vi "Main.vi"(11 "Module Admin":refnum<class "Delacor_lib_QMH_Module Admin.lvclass">) -> ()   [LabVIEW 2020, in "Hardware DAQ.lvlib"]
doc: "This template is based off of the Queued Message Handler design pattern and the Queued Message Handler project template that ships with LabVIEW.\n\nThe main difference is that the queue is private to this module and communication between modules is performed via Broadcast and Request events.\n\nRequest events are wrapped in public API methods and are handled in the Event Handling Loop (EHL) of this VI. Any module can register for Broadcast events sent by this module. The EHL generates messages based on user interface actions.\n\nThe Message Handling Loop (MHL) processes messages generated by the EHL, or by other messages. The messages are string values, so new messages can be added easily to the Message Cases case structure in the MHL. Each message cluster can also provide an optional value for Message Data, which is a variant that can be converted to whatever message-specific data is required.\n_____\nBased on DQMH Project Template 6.0.0.91."
uses:
  Hardware DAQ.lvlib
  <vilib>/Delacor/Delacor QMH/Libraries/Module Admin_class/Delacor_lib_QMH_Module Admin.lvclass
  Module Data--cluster.ctl
  <vilib>/Modbus/master/Modbus Master.lvclass
  Stop Argument--cluster.ctl
  <vilib>/Delacor/Delacor QMH/Libraries/Message Queue_class/Delacor_lib_QMH_Message Queue.lvclass/Delacor_lib_QMH_Message Queue.ctl
  <vilib>/Delacor/Delacor QMH/Libraries/Module Admin_class/Delacor_lib_QMH_Module Admin.lvclass/Delacor_lib_QMH_Module Admin.ctl
  Digital Output 0 Argument--cluster.ctl
  Digital Output 0 (Reply Payload)--cluster.ctl
  Digital Output 1 Argument--cluster.ctl
  Digital Output 1 (Reply Payload)--cluster.ctl
  Digital Output 2 Argument--cluster.ctl
  Digital Output 2 (Reply Payload)--cluster.ctl
  Digital Output 3 Argument--cluster.ctl
  Digital Output 3 (Reply Payload)--cluster.ctl
  <vilib>/Delacor/Delacor QMH/Libraries/Message Queue_class/Delacor_lib_QMH_Enqueue Message (Single).vi
  <vilib>/Delacor/Delacor QMH/Libraries/Module Admin_class/Delacor_lib_QMH_Get External Launch.vi
  <vilib>/DAQmx/read.llb/DAQmx Read (Analog 1D DBL NChan 1Samp).vi
  <vilib>/DAQmx/miscellaneous.llb/DAQmx Fill In Error Info.vi
  <vilib>/Utility/error.llb/Error Cluster From Error Code.vi
  <vilib>/ErrorRing/Error Ring.xnode
  <vilib>/Delacor/Delacor QMH/Libraries/Message Queue_class/Delacor_lib_QMH_Message Queue.lvclass
panel:
  out "Coil values":bool[](array[boolean])
  out "Estado de conexión":bool
  out "Volt":dbl[](array[numeric])
  in  "Update File ini":bool
  in  "Stop System":bool
  in  "Connected System":bool
  in  "Tab Control":enum32{"Adquisición", "Documentación"}(tab)
  out "PLC Logo":bool
  out "Xpress Board":bool
  out "Arduino UNO":bool
  out "NI - 9219":bool
  # "Sistema de Hadrware (DAQ)"
  # "DAQ - 9219"
  # "Arduino UNO"
  # "Xpress Board PIC"
  # "PLC Logo"
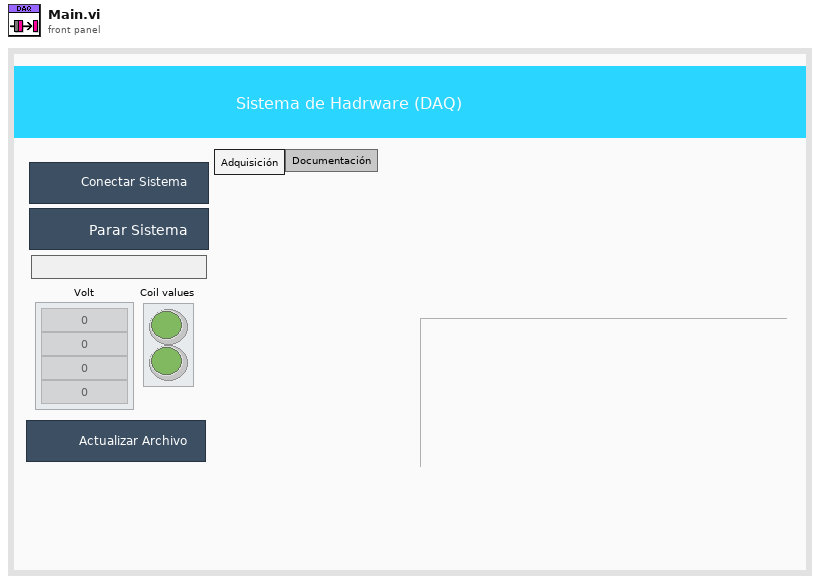
[diagram p1: front panel]
types:
  T1 = typedef "Hardware DAQ.lvlib/Request Events--cluster.ctl" = cluster{"Stop Module":refnum<user-event>, "Show Panel":refnum<user-event>, "Hide Panel":refnum<user-event>, "Get Module Execution Status":refnum<user-event>, "Show Diagram":refnum<user-event>, "Digital Output 0":refnum<user-event>, "Digital Output 1":refnum<user-event>, "Digital Output 2":refnum<user-event>, "Digital Output 3":refnum<user-event>}
  T2 = typedef "Hardware DAQ.lvlib/Module Data--cluster.ctl" = cluster{"File INI":cluster{"Hardware DAQ":cluster{"Hardware":string, "Puerto COM":string, "Task/channels in":string, "Direccion IP PLC":string, "Baudios":string, "Analog Input":string, "Digital Input":string, "Vref Max":string, "Resolución ADC Bits":string}}, "Comunication Hardware DAQ":cluster{"Hardware":enum16{"DAQ9219", "Arduino", "Xpress Board", "PLC Logo", "Default"}, "Status Connected?":bool, "Status File ini?":bool}, "Reference Hardware(s)":cluster{"task out":refnum<k21>, "VISA reference Port":refnum<visa-resource-name>, "TCP master instance":refnum<class "Modbus Master.lvclass">, "#AnalogInput":i32, "#DigitalInput":i32, "Vref Máx":i32, "Resolucion ADC Bits":i32}, "Data Process":cluster{"Volt":dbl[], "Volt DAQ NI9219":dbl[], "coil values":bool[]}}
  T3 = enum32{"invalid lock state", "Not Locked", "Locked (No Password)", "Password-protected"}
  T4 = typedef "Hardware DAQ.lvlib/Stop Argument--cluster.ctl" = cluster{"Origin":string, "Exit via Stop Module Req?":bool, "Wait for Module to stop?":bool}
  T5 = typedef "Hardware DAQ.lvlib/Digital Output 0 Argument--cluster.ctl" = cluster{"Digital Output 0":bool, "Wait Notifier":refnum<notifier>, "wait for reply":bool}
  T6 = typedef "Hardware DAQ.lvlib/Digital Output 1 Argument--cluster.ctl" = cluster{"Digital Output 1":bool, "Wait Notifier":refnum<notifier>, "wait for reply":bool}
  T7 = typedef "Hardware DAQ.lvlib/Digital Output 2 Argument--cluster.ctl" = cluster{"Digital Output 2":bool, "Wait Notifier":refnum<notifier>, "wait for reply":bool}
  T8 = typedef "Hardware DAQ.lvlib/Digital Output 3 Argument--cluster.ctl" = cluster{"Digital Output 3":bool, "Wait Notifier":refnum<notifier>, "wait for reply":bool}
  T9 = enum32{"Invalid", "Standard", "Closed", "Hidden", "Minimized", "Maximized"}
  T10 = enum16{"DAQ9219", "Arduino", "Xpress Board", "PLC Logo", "Default"}
  T11 = typedef "Hardware DAQ.lvlib/Digital Output 0 (Reply Payload)--cluster.ctl" = cluster{"Digital Output 0_I":bool, "error":errorcluster}
  T12 = typedef "Hardware DAQ.lvlib/Digital Output 1 (Reply Payload)--cluster.ctl" = cluster{"Digital Output 1_I":bool, "error":errorcluster}
  T13 = typedef "Hardware DAQ.lvlib/Digital Output 2 (Reply Payload)--cluster.ctl" = cluster{"Digital Output 2_I":bool, "error":errorcluster}
  T14 = typedef "Hardware DAQ.lvlib/Digital Output 3 (Reply Payload)--cluster.ctl" = cluster{"Digital Output 3_I":bool, "error":errorcluster}
  T15 = cluster{"Hardware":string, "Puerto COM":string, "Task/channels in":string, "Direccion IP PLC":string, "Baudios":string, "Analog Input":string, "Digital Input":string, "Vref Max":string, "Resolución ADC Bits":string}
  T16 = cluster{"#Analog Input":i32, "#Digital Input":i32, "Vref Máx":i32, "Resolucion ADC Bits":i32}
  T17 = cluster{"TCP master instance":refnum<class "Modbus Master.lvclass">, "VISA resource":refnum<visa-resource-name>, "task out":refnum<k21>}
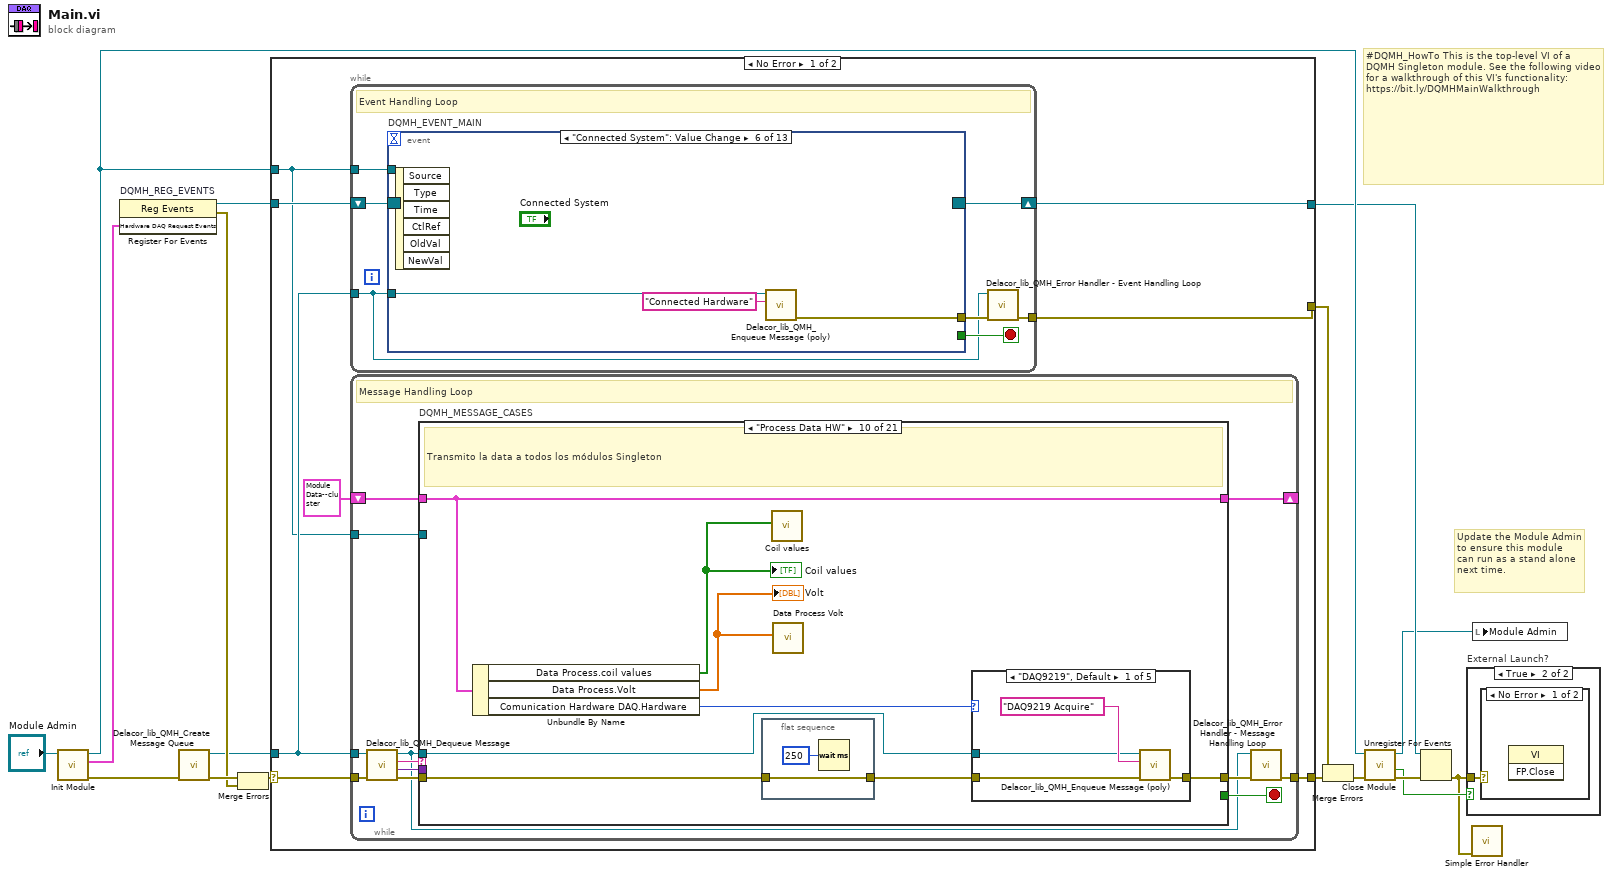
[diagram p0: block diagram]
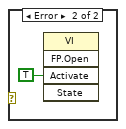
[diagram p3: hidden frame]
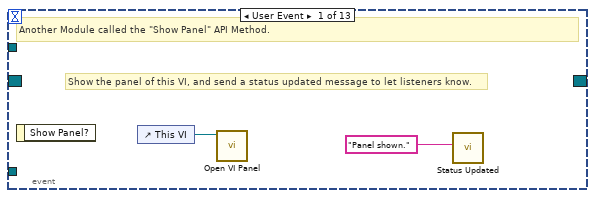
[diagram p4: hidden frame]
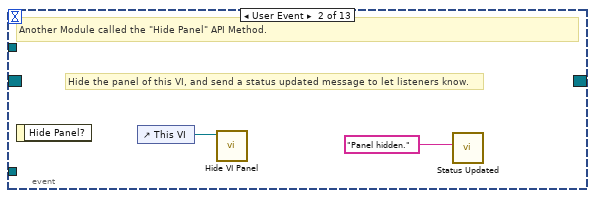
[diagram p5: hidden frame]
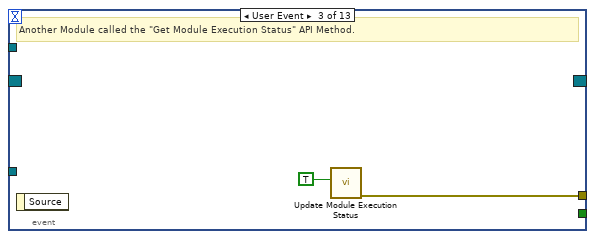
[diagram p6: hidden frame]
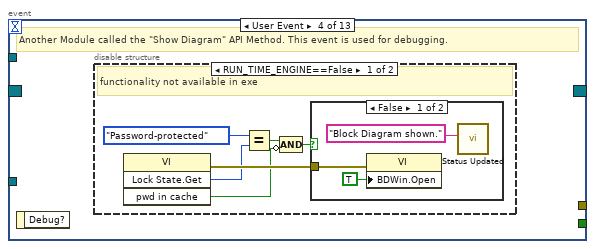
[diagram p7: hidden frame]
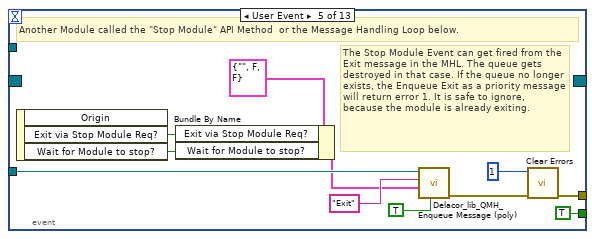
[diagram p10: hidden frame]
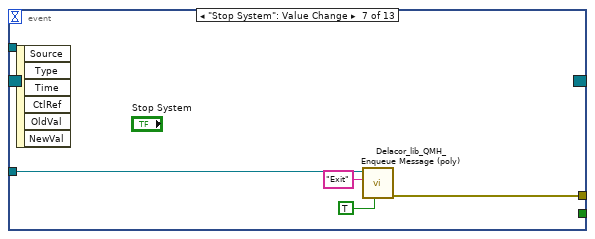
[diagram p11: hidden frame]
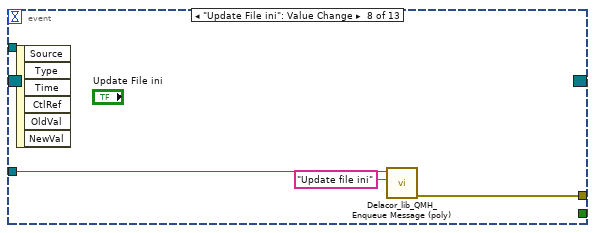
[diagram p12: hidden frame]
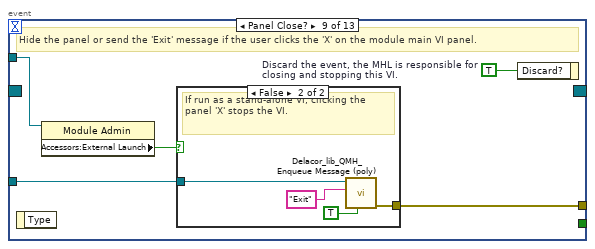
[diagram p13: hidden frame]
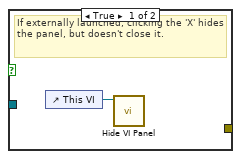
[diagram p14: hidden frame]
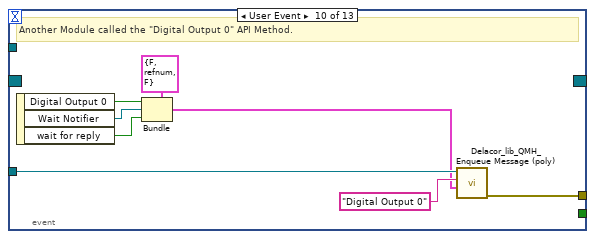
[diagram p15: hidden frame]
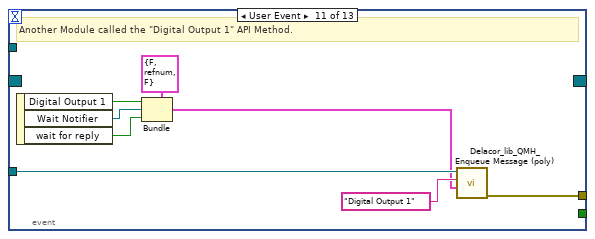
[diagram p16: hidden frame]
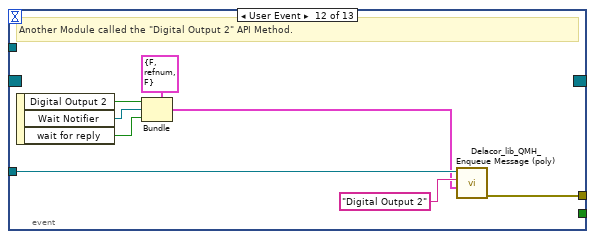
[diagram p17: hidden frame]
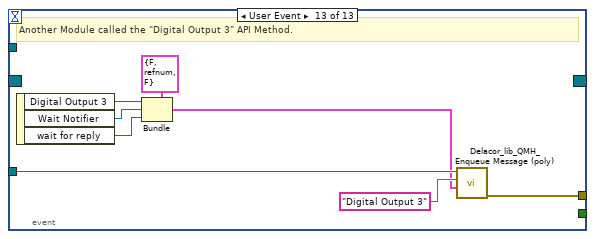
[diagram p18: hidden frame]
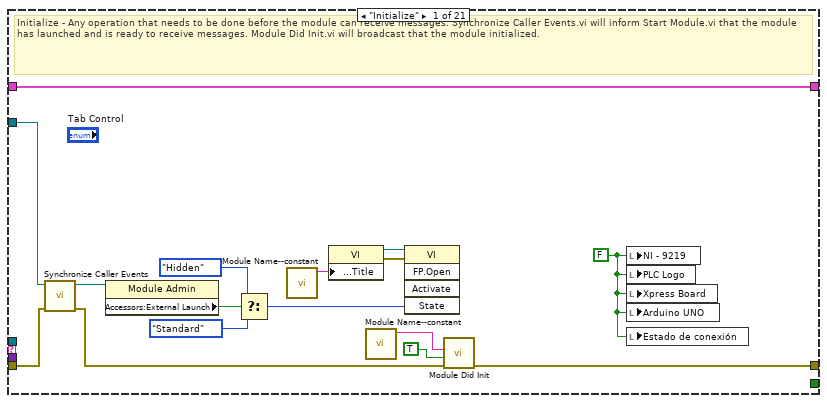
[diagram p19: hidden frame]
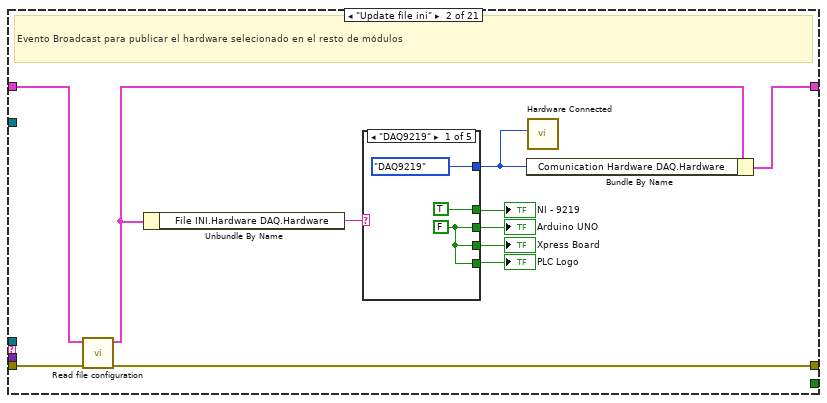
[diagram p20: hidden frame]
diagram:
  # "#DQMH_HowTo This is the top-level VI of a DQMH Singleton module. See the following video for a walkthrough of this VI's functionality: https://bit.ly/DQMHMainWalkthrough"
  # "Update the Module Admin to ensure this module can run as a stand alone next time."
  n1 = call "Init Module.vi"("Singleton Module Admin in"="Module Admin") -> ("error out"=w16:errorcluster, "Hardware DAQ Request Events"=w6:T1, "Singleton Module Admin out"=w9:refnum<class "Delacor_lib_QMH_Module Admin.lvclass">)  [unwired: 8 in]
  n2 = register-events "DQMH_REG_EVENTS"(w6) -> (reference out=w7:refnum<event-registration>, error out=w10:errorcluster)  [unwired: 2 in]
  n3 = call <vilib>:"Delacor_lib_QMH_Create Message Queue.vi"("error in"=w16) -> ("error out"=w12:errorcluster, "Message Queue"=w5:refnum<class "Delacor_lib_QMH_Message Queue.lvclass">)  [unwired: 9 in]
  n4 = Merge Errors(w12, w10) -> (w11:errorcluster)
  n5 = case shown="No Error" w11 {
    selector: w11 -> [w23 w588]
    tunnel: [w25 w587] -> w17
    tunnel: [w22 w593] -> w8
    tunnel: w7 -> [w20 w593]
    tunnel: w5 -> [w19 w586]
    tunnel: [w24 _] -> w14
    tunnel: w9 -> [w18 w589]
    frame No Error {
      n6 = while {
        tunnel: w19 -> [w26]
        shift-right: [w29] -> w22
        shift-left: w20 -> [w30]
        tunnel: [w31] -> w24
        tunnel: w18 -> [w27]
        stop <- w28 stop-if-true
        # "Event Handling Loop"
        n7 = event "DQMH_EVENT_MAIN" shown="[5] \"Connected System\": Value Change" {
          selector: w30 -> [_ _ _ _ _ _ _ _ _ _ _ _ _]
          dyn-events: [_ _ _ _ _ _ _ _ _ _ _ _ _] -> w29
          timeout: _ -> [_ _ _ _ _ _ _ _ _ _ _ _ _]
          tunnel: [_ _ _ _ TRUE ("Discard?") _ _ _ _ _ _ _ _] -> w28
          tunnel: w26 -> [_ _ _ _ w54 w60 w65 w67 w71 w86 w94 w102 w110]
          tunnel: [_ _ w38 _ w57 w61 w62 w68 w73 w79 w87 w95 w103] -> w32
          tunnel: w27 -> [_ _ _ _ _ _ _ _ w70 _ _ _ _]
          event User Event {
            # "Show the panel of this VI, and send a status updated message to let listeners know."
            # "Another Module called the \"Show Panel\" API Method."
            n8 = event-data() -> ()  [unwired: 1 in, 1 out]
            n9 = control-ref of="This VI"() -> (w34:refnum<vi>)
            n10 = call "Open VI Panel.vi"("VI"=w34) -> ()  [unwired: 10 in, 1 out]
            n11 = call "Status Updated.vi"("Status"="Panel shown." ("format string")) -> ()  [unwired: 10 in, 1 out]
          }
          event User Event {
            # "Hide the panel of this VI, and send a status updated message to let listeners know."
            # "Another Module called the \"Hide Panel\" API Method."
            n12 = event-data() -> ()  [unwired: 1 in, 1 out]
            n13 = control-ref of="This VI"() -> (w36:refnum<vi>)
            n14 = call "Hide VI Panel.vi"("VI"=w36) -> ()  [unwired: 10 in, 1 out]
            n15 = call "Status Updated.vi"("Status"="Panel hidden." ("format string")) -> ()  [unwired: 10 in, 1 out]
          }
          event User Event {
            # "Another Module called the \"Get Module Execution Status\" API Method."
            n16 = event-data() -> ()  [unwired: 1 in, 1 out]
            n17 = call "Update Module Execution Status.vi"("Running?"=TRUE) -> ("error out"=w38:errorcluster)  [unwired: 10 in]
          }
          event User Event {
            # "Another Module called the \"Show Diagram\" API Method. This event is used for debugging."
            n18 = event-data() -> ()  [unwired: 1 in, 1 out]
            n19 = disable-structure shown="RUN_TIME_ENGINE==False" {
              frame condition #0 (active) {
                # "functionality not available in exe"
                n20 = invoke class="VI" method="Lock State.Get"() -> (error out=w44:errorcluster, "Get Lock State"=w43:T3, "pwd in cache"=w40:bool)  [unwired: 4 in, 1 out]
                n21 = Equal?(x=T3."Password-protected", y=w43) -> (x = y?=w41:bool)
                n22 = Compound Arithmetic op=AND(w41, invert w40) -> (w39:bool)
                n23 = case shown="False" w39 {
                  tunnel: w44 -> [w47 _]
                  frame False {
                    n24 = property class="VI"(error in=w47, "BDWin.Open"=TRUE ("Block Diagram Window:Open")) -> ()  [unwired: 1 in, 2 out]
                    n25 = call "Status Updated.vi"("Status"="Block Diagram shown." ("format string")) -> ()  [unwired: 10 in, 1 out]
                  }
                  frame True {
                    # "Password-protected VI, and the password is not in the cache. Do not show the diagram."
                  }
                }
              }
              frame condition #1 {
              }
            }
          }
          event User Event {
            # "The Stop Module Event can get fired from the Exit message in the MHL. The queue gets destroyed in that case. If the queue no longer exists, the Enqueue Exit as a priority message will return error 1. It is safe to ignore, because the module is already exiting."
            # "Another Module called the \"Stop Module\" API Method  or the Message Handling Loop below."
            n26 = event-data() -> ("Exit via Stop Module Req?"=w50:bool, "Wait for Module to stop?"=w49:bool)  [unwired: 1 in, 1 out]
            n27 = Bundle By Name(cluster=T4 {"Origin"="", "Exit via Stop Module Req?"=FALSE, "Wait for Module to stop?"=FALSE} ("Stop Argument"), "Exit via Stop Module Req?"=w50, "Wait for Module to stop?"=w49) -> (w48:T4)
            n28 = call-poly <vilib>:"Delacor_lib_QMH_Enqueue Message (poly).vi"("Priority Message? (F)"=TRUE, "Message Data"=w48, "Message"="Exit", "Message Queue in"=w54) -> ("error out"=w58:errorcluster)  [unwired: 6 in, 1 out]
            n29 = call <vilib>:"Clear Errors.vi"("error in (no error)"=w58, "specific error code to clear (0: all)"=1) -> ("error out"=w57:errorcluster)  [unwired: 4 in, 1 out]
          }
          event "Connected System": Value Change {
            n30 = event-data() -> ()  [unwired: 1 in, 6 out]
            n31 = call-poly <vilib>:"Delacor_lib_QMH_Enqueue Message (poly).vi"("Message"="Connected Hardware", "Message Queue in"=w60) -> ("error out"=w61:errorcluster)  [unwired: 8 in, 1 out]
          }
          event "Stop System": Value Change {
            n32 = event-data() -> ()  [unwired: 1 in, 6 out]
            n33 = call-poly <vilib>:"Delacor_lib_QMH_Enqueue Message (poly).vi"("Priority Message? (F)"=TRUE, "Message"="Exit", "Message Queue in"=w65) -> ("error out"=w62:errorcluster)  [unwired: 7 in, 1 out]
          }
          event "Update File ini": Value Change {
            n34 = event-data() -> ()  [unwired: 1 in, 6 out]
            n35 = call-poly <vilib>:"Delacor_lib_QMH_Enqueue Message (poly).vi"("Message"="Update file ini", "Message Queue in"=w67) -> ("error out"=w68:errorcluster)  [unwired: 8 in, 1 out]
          }
          event Panel Close? {
            w72 = TRUE  # Discard the event, the MHL is responsible for closing and stopping this VI.
            # "Hide the panel or send the 'Exit' message if the user clicks the 'X' on the module main VI panel."
            n36 = event-data() -> ()  [unwired: 1 in, 1 out]
            n37 = property class="Module Admin"(reference=w70) -> ("Accessors:External Launch"=w69:bool)  [unwired: 1 in, 2 out]
            n38 = case shown="False" w69 {
              tunnel: w71 -> [_ w77]
              tunnel: [_ w78] -> w73
              frame True {
                # "If externally launched, clicking the 'X' hides the panel, but doesn't close it."
                n39 = control-ref of="This VI"() -> (w74:refnum<vi>)
                n40 = call "Hide VI Panel.vi"("VI"=w74) -> ()  [unwired: 10 in, 1 out]
              }
              frame False {
                # "If run as a stand-alone VI, clicking the panel 'X' stops the VI."
                n41 = call-poly <vilib>:"Delacor_lib_QMH_Enqueue Message (poly).vi"("Priority Message? (F)"=TRUE, "Message"="Exit", "Message Queue in"=w77) -> ("error out"=w78:errorcluster)  [unwired: 7 in, 1 out]
              }
            }
            n42 = event-data("Discard?"=w72) -> ()  [unwired: 1 in, 1 out]
          }
          event User Event {
            # "Another Module called the \"Digital Output 0\" API Method."
            n43 = event-data() -> ("Digital Output 0"=w82:bool, "Wait Notifier"=w81:refnum<notifier>, "wait for reply"=w80:bool)  [unwired: 1 in]
            n44 = Bundle(cluster=T5 {"Digital Output 0"=FALSE, "Wait Notifier"=refnum, "wait for reply"=FALSE} ("Digital Output 0 Argument"), "Digital Output 0"=w82, "Wait Notifier"=w81, "wait for reply"=w80) -> (w83:T5)
            n45 = call-poly <vilib>:"Delacor_lib_QMH_Enqueue Message (poly).vi"("Message Data"=w83, "Message"="Digital Output 0", "Message Queue in"=w86) -> ("error out"=w79:errorcluster)  [unwired: 7 in, 1 out]
          }
          event User Event {
            # "Another Module called the \"Digital Output 1\" API Method."
            n46 = event-data() -> ("Digital Output 1"=w90:bool, "Wait Notifier"=w89:refnum<notifier>, "wait for reply"=w88:bool)  [unwired: 1 in]
            n47 = Bundle(cluster=T6 {"Digital Output 1"=FALSE, "Wait Notifier"=refnum, "wait for reply"=FALSE} ("Digital Output 1 Argument"), "Digital Output 1"=w90, "Wait Notifier"=w89, "wait for reply"=w88) -> (w91:T6)
            n48 = call-poly <vilib>:"Delacor_lib_QMH_Enqueue Message (poly).vi"("Message Data"=w91, "Message"="Digital Output 1", "Message Queue in"=w94) -> ("error out"=w87:errorcluster)  [unwired: 7 in, 1 out]
          }
          event User Event {
            # "Another Module called the \"Digital Output 2\" API Method."
            n49 = event-data() -> ("Digital Output 2"=w98:bool, "Wait Notifier"=w97:refnum<notifier>, "wait for reply"=w96:bool)  [unwired: 1 in]
            n50 = Bundle(cluster=T7 {"Digital Output 2"=FALSE, "Wait Notifier"=refnum, "wait for reply"=FALSE} ("Digital Output 2 Argument"), "Digital Output 2"=w98, "Wait Notifier"=w97, "wait for reply"=w96) -> (w99:T7)
            n51 = call-poly <vilib>:"Delacor_lib_QMH_Enqueue Message (poly).vi"("Message Data"=w99, "Message"="Digital Output 2", "Message Queue in"=w102) -> ("error out"=w95:errorcluster)  [unwired: 7 in, 1 out]
          }
          event User Event {
            # "Another Module called the \"Digital Output 3\" API Method."
            n52 = event-data() -> ("Digital Output 3"=w106:bool, "Wait Notifier"=w105:refnum<notifier>, "wait for reply"=w104:bool)  [unwired: 1 in]
            n53 = Bundle(cluster=T8 {"Digital Output 3"=FALSE, "Wait Notifier"=refnum, "wait for reply"=FALSE} ("Digital Output 3 Argument"), "Digital Output 3"=w106, "Wait Notifier"=w105, "wait for reply"=w104) -> (w107:T8)
            n54 = call-poly <vilib>:"Delacor_lib_QMH_Enqueue Message (poly).vi"("Message Data"=w107, "Message"="Digital Output 3", "Message Queue in"=w110) -> ("error out"=w103:errorcluster)  [unwired: 7 in, 1 out]
          }
        }
        n55 = call-dynamic "Delacor_lib_QMH_Error Handler - Event Handling Loop.vi"("error in"=w32, "Message Queue in"=w26) -> ("dup error in"=w31:errorcluster)  [unwired: 8 in, 1 out]
      }
      n56 = while {
        tunnel: w19 -> [w113]
        shift-right: [w117] -> _
        shift-left: T2 {"File INI"={"Hardware DAQ"={"Hardware"="", "Puerto COM"="", "Task/channels in"="", "Direccion IP PLC"="", "Baudios"="", "Analog Input"="", "Digital Input"="", "Vref Max"="", "Resolución ADC Bits"=""}}, "Comunication Hardware DAQ"={"Hardware"=enum."DAQ9219", "Status Connected?"=FALSE, "Status File ini?"=FALSE}, "Reference Hardware(s)"={"task out"="", "VISA reference Port"="", "TCP master instance"=refnum, "#AnalogInput"=0, "#DigitalInput"=0, "Vref Máx"=0, "Resolucion ADC Bits"=0}, "Data Process"={"Volt"=[], "Volt DAQ NI9219"=[], "coil values"=[]}} ("Data Cluster") -> [w118]
        tunnel: w23 -> [w121]
        tunnel: [w119] -> w25
        tunnel: w18 -> [w111]
        stop <- w116 stop-if-true
        # "Message Handling Loop"
        n57 = call-dynamic "Delacor_lib_QMH_Dequeue Message.vi"("error in"=w121, "Message Queue in"=w113) -> ("error out"=w120:errorcluster, "Message Data"=w114:variant, "Message"=w115:string, "Message Queue out"=w112:refnum<class "Delacor_lib_QMH_Message Queue.lvclass">)  [unwired: 6 in]
        n58 = case "DQMH_MESSAGE_CASES" shown="\"Process Data HW\"" w115 {
          selector: w115 -> [_ _ _ _ _ _ _ _ _ _ _ _ _ _ _ _ _ _ _ _ w573]
          tunnel: w112 -> [_ _ w179 w187 w208 w221 w251 w278 w284 w298 _ _ _ _ _ _ _ _ w540 w566 _]
          tunnel: w120 -> [w137 w149 w178 w185 w216 w227 w257 w280 w294 w299 w323 w342 w391 w440 w489 w522 w524 w529 w546 w571 w575]
          tunnel: [w135 w139 w180 w186 w207 w220 w250 w279 w283 w297 w323 w328 w374 w422 w471 w521 w524 w528 w537 w568 w576] -> w122
          tunnel: w118 -> [w124 w148 w183 w189 w215 w231 w261 w282 w290 w302 w322 w330 w383 w432 w481 w520 w523 w526 w542 w554 w574]
          tunnel: [w124 w145 w182 w189 w211 w222 w252 w282 w287 w302 w322 w327 w382 w431 w480 w520 w523 w526 w542 w554 w574] -> w117
          tunnel: [_ _ _ _ _ _ _ _ _ _ _ _ _ _ _ _ _ _ _ w565 _] -> w116
          tunnel: w114 -> [_ _ _ _ _ _ _ _ _ _ _ w341 w390 w439 w488 _ _ _ w541 w564 _]
          tunnel: w111 -> [w128 _ _ _ _ _ _ _ _ _ _ _ _ _ _ _ _ _ w539 w559 _]
          frame "Initialize" {
            w123 = FALSE ("PLC Logo")
            # "Initialize - Any operation that needs to be done before the module can receive messages. Synchronize Caller Events.vi will inform Start Module.vi that the module has launched and is ready to receive messages. Module Did Init.vi will broadcast that the module initialized."
            n59 = call "Synchronize Caller Events.vi"("error in (no error)"=w137, "Singleton Module Admin in"=w128) -> ("error out"=w136:errorcluster, "Singleton Module Admin out"=w125:refnum<class "Delacor_lib_QMH_Module Admin.lvclass">)  [unwired: 8 in]
            n60 = property class="Module Admin"(reference=w125) -> ("Accessors:External Launch"=w132:bool)  [unwired: 1 in, 2 out]
            n61 = Select(t=T9."Hidden" ("State"), s=w132, f=T9."Standard" ("State")) -> (s? t:f=w129:T9)
            n62 = call "Module Name--constant.vi"() -> ("Module Name"=w134:string)  [unwired: 11 in]
            n63 = property class="VI"("Front Panel.Title"=w134) -> (reference out=w133:refnum<vi>, error out=w138:errorcluster)  [unwired: 2 in]
            n64 = call "Module Name--constant.vi"() -> ("Module Name"=w126:string)  [unwired: 11 in]
            n65 = invoke class="VI" method="FP.Open"(reference=w133, error in=w138, "State"=w129) -> ()  [unwired: 2 in, 5 out]
            n66 = call "Module Did Init.vi"("error in (no error)"=w136, "Initialized?"=TRUE, "Origin"=w126) -> ("error out"=w135:errorcluster)  [unwired: 8 in]
            n67 = local write "NI - 9219"(w123) -> ()
            n68 = local write "PLC Logo"(w123) -> ()
            n69 = local write "Xpress Board"(w123) -> ()
            n70 = local write "Arduino UNO"(w123) -> ()
            n71 = local write "Estado de conexión"(w123) -> ()
          }
          frame "Update file ini" {
            # "Evento Broadcast para publicar el hardware selecionado en el resto de módulos"
            n72 = call "Read file configuration.vi"("error in (no error)"=w149, "Data Cluster"=w148) -> ("error out"=w139:errorcluster, "Data Cluster out"=w146:T2)  [unwired: 8 in]
            n73 = Unbundle By Name(w146) -> ("File INI.Hardware DAQ.Hardware"=w147:string)
            n74 = case shown="\"DAQ9219\"" w147 {
              tunnel: [TRUE ("NI - 9219") w154 w157 w160 w163] -> w143
              tunnel: [w151 TRUE ("Arduino UNO") w157 w160 w163] -> w142
              tunnel: [w151 w154 TRUE ("Arduino UNO") w160 w163] -> w141
              tunnel: [w151 w154 w157 TRUE ("Arduino UNO") w163] -> w140
              tunnel: [T10."DAQ9219" T10."Arduino" T10."Xpress Board" T10."PLC Logo" T10."Default"] -> w144
              frame "DAQ9219" {
                w151 = FALSE ("Arduino UNO")
              }
              frame "Arduino" {
                w154 = FALSE ("NI - 9219")
              }
              frame "Xpress Board" {
                w157 = FALSE ("NI - 9219")
              }
              frame "PLC" {
                w160 = FALSE ("NI - 9219")
              }
              frame "Default", Default {
                w163 = FALSE ("NI - 9219")
              }
            }
            "NI - 9219" <- w143
            "Arduino UNO" <- w142
            "Xpress Board" <- w141
            "PLC Logo" <- w140
            n75 = Bundle By Name(cluster=w146, "Comunication Hardware DAQ.Hardware"=w144) -> (w145:T2)
            n76 = call "Hardware Connected.vi"("Hardware Connected"=w144) -> ()  [unwired: 10 in, 1 out]
          }
          frame "Connected Hardware" {
            n77 = Unbundle By Name(w183) -> ("File INI.Hardware DAQ"=w176:T15, "Comunication Hardware DAQ.Hardware"=w177:T10)
            n78 = call "Select Hardware.vi"("error in (no error)"=w178, "Hardware"=w177, "File INI.Hardware DAQ"=w176) -> ("error out"=w164:errorcluster, "#Parametros HW"=w171:T16, "Reference HW"=w175:T17)  [unwired: 6 in]
            n79 = Unbundle By Name(w171) -> ("#Analog Input"=w170:i32, "#Digital Input"=w169:i32, "Vref Máx"=w168:i32, "Resolucion ADC Bits"=w167:i32)
            n80 = Unbundle By Name(w175) -> ("TCP master instance"=w174:refnum<class "Modbus Master.lvclass">, "task out"=w173:refnum<k21>, "VISA resource"=w172:refnum<visa-resource-name>)
            n81 = Unbundle By Name(w164) -> ("status"=w166:bool)
            n82 = Not(x=w166) -> (.not. x?=w165:bool)
            n83 = Bundle By Name(cluster=w183, "Reference Hardware(s).TCP master instance"=w174, "Reference Hardware(s).task out"=w173, "Reference Hardware(s).VISA reference Port"=w172, "Reference Hardware(s).#AnalogInput"=w170, "Reference Hardware(s).#DigitalInput"=w169, "Reference Hardware(s).Vref Máx"=w168, "Reference Hardware(s).Resolucion ADC Bits"=w167, "Comunication Hardware DAQ.Status Connected?"=w165) -> (w182:T2)
            n84 = call-poly <vilib>:"Delacor_lib_QMH_Enqueue Message (poly).vi"("error in"=w164, "Message"="Update HMI User", "Message Queue in"=w179) -> ("error out"=w180:errorcluster)  [unwired: 7 in, 1 out]
          }
          frame "Update HMI User" {
            n85 = Unbundle By Name(w189) -> ("Comunication Hardware DAQ.Status Connected?"=→"Estado de conexión":bool, "Comunication Hardware DAQ.Hardware"=w188:T10)
            n86 = case shown="\"DAQ9219\", Default" w188 {
              tunnel: w187 -> [w192 w196 w200 w204 _]
              tunnel: [w191 w195 w199 w203 w206] -> w186
              tunnel: w185 -> [w190 w194 w198 w202 w206]
              frame "DAQ9219", Default {
                n87 = call-poly <vilib>:"Delacor_lib_QMH_Enqueue Message (poly).vi"("error in"=w190, "Message"="DAQ9219 Acquire", "Message Queue in"=w192) -> ("error out"=w191:errorcluster)  [unwired: 7 in, 1 out]
              }
              frame "Arduino" {
                n88 = call-poly <vilib>:"Delacor_lib_QMH_Enqueue Message (poly).vi"("error in"=w194, "Message"="Arduino Acquire", "Message Queue in"=w196) -> ("error out"=w195:errorcluster)  [unwired: 7 in, 1 out]
              }
              frame "Xpress Board" {
                n89 = call-poly <vilib>:"Delacor_lib_QMH_Enqueue Message (poly).vi"("error in"=w198, "Message"="Xpress Board Acquire", "Message Queue in"=w200) -> ("error out"=w199:errorcluster)  [unwired: 7 in, 1 out]
              }
              frame "PLC Logo" {
                n90 = call-poly <vilib>:"Delacor_lib_QMH_Enqueue Message (poly).vi"("error in"=w202, "Message"="PLC Acquire", "Message Queue in"=w204) -> ("error out"=w203:errorcluster)  [unwired: 7 in, 1 out]
              }
              frame "Default" {
              }
            }
          }
          frame "DAQ9219 Acquire" {
            n91 = Unbundle By Name(w215) -> ("Reference Hardware(s).task out"=w217:refnum<k21>)
            n92 = call-poly <vilib>:"DAQmx Read.vi"("task/channels in"=w217, "timeout"=1000.0, "error in"=w216) -> ("task out"=w214:refnum<k21>, "data"=w213:dbl[], "error out"=w209:errorcluster)  [unwired: 10 in]
            n93 = Bundle By Name(cluster=w215, "Reference Hardware(s).task out"=w214, "Data Process.Volt"=w213) -> (w211:T2)
            n94 = call-poly <vilib>:"Delacor_lib_QMH_Enqueue Message (poly).vi"("error in"=w209, "Message"="Process Data HW", "Message Queue in"=w208) -> ("error out"=w207:errorcluster)  [unwired: 7 in, 1 out]
          }
          frame "Arduino Acquire" {
            w226 = enum16{"AI-0", "AI-1", "AI-2", "AI-3"}[] [enum."AI-0", enum."AI-1", enum."AI-2", enum."AI-3"] items=["AI-0", "AI-1", "AI-2", "AI-3"]
            n95 = Unbundle By Name(w231) -> ("Reference Hardware(s).VISA reference Port"=w230:refnum<visa-resource-name>, "Reference Hardware(s).#AnalogInput"=w225:i32, "Reference Hardware(s).Vref Máx"=w229:i32, "Reference Hardware(s).Resolucion ADC Bits"=w228:i32)  [unwired: 1 out]
            n96 = for {
              N: w225 -> [_]
              tunnel: w230 -> [w247]
              tunnel: w229 -> [w244]
              tunnel: w228 -> [w243]
              tunnel: w227 -> [w246]
              tunnel: w226 -> [w245] mode=indexing
              tunnel: [w242] -> w218
              tunnel: [w241] -> w224
              tunnel: [w240] -> w223 mode=indexing
              n97 = call "Read Analog Input.vi"("VISA Refnum in"=w247, "#Pin analogico"=w245, "Vref Máx"=w244, "Resolucion ADC Bits"=w243, "error in (no error)"=w246) -> ("VISA Refnum out"=w241:refnum<visa-resource-name>, "Volt"=w240:dbl, "error out"=w242:errorcluster)  [unwired: 8 in]
            }
            n98 = Unbundle By Name(w218) -> ("code"=w219:i32)
            n99 = Bundle By Name(cluster=w231, "Reference Hardware(s).VISA reference Port"=w224, "Data Process.Volt"=w223) -> (w222:T2)
            n100 = case shown="1023" w219 {
              tunnel: w221 -> [w232 w238]
              tunnel: [w233 w237] -> w220
              tunnel: w218 -> [w234 w236]
              frame 1023 {
                n101 = call-poly <vilib>:"Delacor_lib_QMH_Enqueue Message (poly).vi"("error in"=w234, "Message"="Exit", "Message Queue in"=w232) -> ("error out"=w233:errorcluster)  [unwired: 7 in, 1 out]
              }
              frame 1, Default {
                n102 = call-poly <vilib>:"Delacor_lib_QMH_Enqueue Message (poly).vi"("error in"=w236, "Message"="Process Data HW", "Message Queue in"=w238) -> ("error out"=w237:errorcluster)  [unwired: 7 in, 1 out]
              }
            }
          }
          frame "Xpress Board Acquire" {
            w256 = enum16{"AI-0", "AI-1", "AI-2", "AI-3"}[] [enum."AI-0", enum."AI-1", enum."AI-2", enum."AI-3"] items=["AI-0", "AI-1", "AI-2", "AI-3"]
            n103 = Unbundle By Name(w261) -> ("Reference Hardware(s).VISA reference Port"=w260:refnum<visa-resource-name>, "Reference Hardware(s).#AnalogInput"=w255:i32, "Reference Hardware(s).Vref Máx"=w259:i32, "Reference Hardware(s).Resolucion ADC Bits"=w258:i32)  [unwired: 1 out]
            n104 = for {
              N: w255 -> [_]
              tunnel: w260 -> [w277]
              tunnel: w259 -> [w274]
              tunnel: w258 -> [w273]
              tunnel: w257 -> [w276]
              tunnel: w256 -> [w275] mode=indexing
              tunnel: [w272] -> w248
              tunnel: [w271] -> w254
              tunnel: [w270] -> w253 mode=indexing
              n105 = call "Read Analog Input.vi"("VISA Refnum in"=w277, "#Pin analogico"=w275, "Vref Máx"=w274, "Resolucion ADC Bits"=w273, "error in (no error)"=w276) -> ("VISA Refnum out"=w271:refnum<visa-resource-name>, "Volt"=w270:dbl, "error out"=w272:errorcluster)  [unwired: 8 in]
            }
            n106 = Unbundle By Name(w248) -> ("code"=w249:i32)
            n107 = Bundle By Name(cluster=w261, "Reference Hardware(s).VISA reference Port"=w254, "Data Process.Volt"=w253) -> (w252:T2)
            n108 = case shown="Default" w249 {
              tunnel: w251 -> [w262 w268]
              tunnel: [w263 w267] -> w250
              tunnel: w248 -> [w264 w266]
              frame 1023 {
                n109 = call-poly <vilib>:"Delacor_lib_QMH_Enqueue Message (poly).vi"("error in"=w264, "Message"="Exit", "Message Queue in"=w262) -> ("error out"=w263:errorcluster)  [unwired: 7 in, 1 out]
              }
              frame Default {
                n110 = call-poly <vilib>:"Delacor_lib_QMH_Enqueue Message (poly).vi"("error in"=w266, "Message"="Process Data HW", "Message Queue in"=w268) -> ("error out"=w267:errorcluster)  [unwired: 7 in, 1 out]
              }
            }
          }
          frame "PLC Acquire" {
            n111 = call-poly <vilib>:"Delacor_lib_QMH_Enqueue Message (poly).vi"("error in"=w280, "Message"="Read Digital Inputs", "Message Queue in"=w278) -> ("error out"=w279:errorcluster)  [unwired: 7 in, 1 out]
          }
          frame "Read Digital Inputs" {
            n112 = Unbundle By Name(w290) -> ("Reference Hardware(s).TCP master instance"=w293:refnum<class "Modbus Master.lvclass">)
            n113 = call-dynamic "Read Coils.vi"("error in (no error)"=w294, "number of coils"=u16 4, "starting address"=u16 0, "Modbus master in"=w293) -> ("error out"=w285:errorcluster, "coil values"=w288:bool[], "Modbus master out"=w289:refnum<class "Modbus Master.lvclass">)  [unwired: 5 in]
            n114 = Bundle By Name(cluster=w290, "Reference Hardware(s).TCP master instance"=w289, "Data Process.coil values"=w288) -> (w287:T2)
            n115 = call-poly <vilib>:"Delacor_lib_QMH_Enqueue Message (poly).vi"("error in"=w285, "Message"="Process Data HW", "Message Queue in"=w284) -> ("error out"=w283:errorcluster)  [unwired: 7 in, 1 out]
          }
          frame "Process Data HW" {
            # "Transmito la data a todos los módulos Singleton"
            n116 = Unbundle By Name(w302) -> ("Data Process.coil values"=w295:bool[], "Data Process.Volt"=w296:dbl[], "Comunication Hardware DAQ.Hardware"=w301:T10)
            "Volt" <- w296
            "Coil values" <- w295
            n117 = flat-sequence {
              tunnel: [w304] -> w300
              tunnel: w299 -> [w304]
              frame #0 {
                n118 = Wait (ms)(milliseconds to wait=u32 250) -> ()  [unwired: 1 out]
              }
            }
            n119 = call "Coil values.vi"("Data Process.coil values"=w295) -> ()  [unwired: 10 in, 1 out]
            n120 = call "Data Process Volt.vi"("Data Process.Volt"=w296) -> ()  [unwired: 10 in, 1 out]
            n121 = case shown="\"DAQ9219\", Default" w301 {
              tunnel: w298 -> [w307 w311 w315 w319 _]
              tunnel: [w306 w310 w314 w318 w321] -> w297
              tunnel: w300 -> [w305 w309 w313 w317 w321]
              frame "DAQ9219", Default {
                n122 = call-poly <vilib>:"Delacor_lib_QMH_Enqueue Message (poly).vi"("error in"=w305, "Message"="DAQ9219 Acquire", "Message Queue in"=w307) -> ("error out"=w306:errorcluster)  [unwired: 7 in, 1 out]
              }
              frame "Arduino" {
                n123 = call-poly <vilib>:"Delacor_lib_QMH_Enqueue Message (poly).vi"("error in"=w309, "Message"="Arduino Acquire", "Message Queue in"=w311) -> ("error out"=w310:errorcluster)  [unwired: 7 in, 1 out]
              }
              frame "Xpress Board" {
                n124 = call-poly <vilib>:"Delacor_lib_QMH_Enqueue Message (poly).vi"("error in"=w313, "Message"="Xpress Board Acquire", "Message Queue in"=w315) -> ("error out"=w314:errorcluster)  [unwired: 7 in, 1 out]
              }
              frame "PLC Logo" {
                n125 = call-poly <vilib>:"Delacor_lib_QMH_Enqueue Message (poly).vi"("error in"=w317, "Message"="PLCAcquire", "Message Queue in"=w319) -> ("error out"=w318:errorcluster)  [unwired: 7 in, 1 out]
              }
              frame "Default" {
              }
            }
          }
          frame "---Module Specific---" {
            # "Separator -- The following cases handle messages specific to this Module."
          }
          frame "Digital Output 0" {
            # "Digital Output 0 to Hardware"
            n126 = Variant To Data(error in=w342, type=T5 {"Digital Output 0"=FALSE, "Wait Notifier"=refnum, "wait for reply"=FALSE} ("Digital Output 0 Argument"), Variant=w341) -> (data=w339:T5, error out=w334:errorcluster)
            n127 = Unbundle By Name(w330) -> ("Reference Hardware(s).TCP master instance"=w325:refnum<class "Modbus Master.lvclass">, "Reference Hardware(s).VISA reference Port"=w333:refnum<visa-resource-name>, "Comunication Hardware DAQ.Hardware"=w326:T10)
            n128 = Unbundle By Name(w339) -> ("Digital Output 0"=w332:bool, "Wait Notifier"=w338:refnum<notifier>, "wait for reply"=w337:bool)
            n129 = case shown="\"Xpress Board\"" w326 {
              tunnel: w334 -> [w346 w354 w362 w370]
              tunnel: w333 -> [w344 w353 w361 w363]
              tunnel: w332 -> [w345 w351 w359 w369]
              tunnel: [w345 w350 w358 w364] -> w331
              tunnel: [w344 w349 w357 w363] -> w329
              tunnel: [w346 w348 w356 w366] -> w328
              tunnel: w325 -> [w343 w347 w355 w368]
              tunnel: [w343 w347 w355 w365] -> w324
              frame "DAQ9219", Default {
                # "No hay nada"
              }
              frame "Arduino" {
                n130 = call "Write Digital Output.vi"("error in (no error)"=w354, "State"=w351, "#Pin Digital Out"=enum16{"DO-0", "DO-1", "DO-2", "DO-3"}."DO-0", "VISA reference in"=w353) -> ("error out"=w348:errorcluster, "State dispare?"=w350:bool, "VISA reference out"=w349:refnum<visa-resource-name>)  [unwired: 5 in]
              }
              frame "Xpress Board" {
                n131 = call "Write Digital Output.vi"("error in (no error)"=w362, "State"=w359, "#Pin Digital Out"=enum16{"DO-0", "DO-1", "DO-2", "DO-3"}."DO-0", "VISA reference in"=w361) -> ("error out"=w356:errorcluster, "State dispare?"=w358:bool, "VISA reference out"=w357:refnum<visa-resource-name>)  [unwired: 5 in]
              }
              frame "PLC Logo" {
                n132 = call "Digital Output 0-10V.vi"("error in (no error)"=w370, "State"=w369, "#Pin 0-10V"=enum16{"DO-0", "DO-1", "DO-2", "DO-3"}."DO-0", "Modbus Master in"=w368) -> ("error out"=w366:errorcluster, "State Send?"=w364:bool, "Modbus master out"=w365:refnum<class "Modbus Master.lvclass">)  [unwired: 5 in]
              }
            }
            n133 = Bundle By Name(cluster=w330, "Reference Hardware(s).TCP master instance"=w324, "Reference Hardware(s).VISA reference Port"=w329) -> (w327:T2)
            n134 = Bundle By Name(cluster=T11 {"Digital Output 0_I"=FALSE, "error"={"status"=FALSE, "code"=0, "source"=""}} ("Digital Output 0 (Reply Payload)"), "Digital Output 0_I"=w331, "error"=w328) -> (w336:T11)
            n135 = case shown="True" w337 {
              tunnel: w338 -> [_ w372]
              tunnel: w336 -> [_ w371]
              frame False {
              }
              frame True {
                n136 = Send Notification(notification=w371, notifier=w372) -> ()  [unwired: 1 in, 2 out]
              }
            }
          }
          frame "Digital Output 1" {
            # "Digital Output 1 to Hardware"
            n137 = Variant To Data(error in=w391, type=T6 {"Digital Output 1"=FALSE, "Wait Notifier"=refnum, "wait for reply"=FALSE} ("Digital Output 1 Argument"), Variant=w390) -> (data=w388:T6, error out=w381:errorcluster)
            n138 = Unbundle By Name(w383) -> ("Reference Hardware(s).TCP master instance"=w378:refnum<class "Modbus Master.lvclass">, "Reference Hardware(s).VISA reference Port"=w379:refnum<visa-resource-name>, "Comunication Hardware DAQ.Hardware"=w380:T10)
            n139 = Unbundle By Name(w388) -> ("Digital Output 1"=w373:bool, "Wait Notifier"=w387:refnum<notifier>, "wait for reply"=w386:bool)
            n140 = case shown="\"PLC Logo\"" w380 {
              tunnel: [FALSE ("State Send?") w402 w410 w416] -> w375
              tunnel: [w393 w401 w409 w413] -> w376
              tunnel: [w395 w400 w408 w418] -> w374
              tunnel: [w392 w399 w405 w417] -> w377
              tunnel: w381 -> [w395 w398 w407 w415]
              tunnel: w379 -> [w393 w396 w406 w413]
              tunnel: w378 -> [w392 w399 w405 w412]
              tunnel: w373 -> [_ w397 w404 w414]
              frame "DAQ9219", Default {
                # "No hay nada"
              }
              frame "Arduino" {
                n141 = call "Write Digital Output.vi"("error in (no error)"=w398, "State"=w397, "#Pin Digital Out"=enum16{"DO-0", "DO-1", "DO-2", "DO-3"}."DO-1", "VISA reference in"=w396) -> ("error out"=w400:errorcluster, "State dispare?"=w402:bool, "VISA reference out"=w401:refnum<visa-resource-name>)  [unwired: 5 in]
              }
              frame "Xpress Board" {
                n142 = call "Write Digital Output.vi"("error in (no error)"=w407, "State"=w404, "#Pin Digital Out"=enum16{"DO-0", "DO-1", "DO-2", "DO-3"}."DO-1", "VISA reference in"=w406) -> ("error out"=w408:errorcluster, "State dispare?"=w410:bool, "VISA reference out"=w409:refnum<visa-resource-name>)  [unwired: 5 in]
              }
              frame "PLC Logo" {
                n143 = call "Digital Output 0-10V.vi"("error in (no error)"=w415, "State"=w414, "#Pin 0-10V"=enum16{"DO-0", "DO-1", "DO-2", "DO-3"}."DO-1", "Modbus Master in"=w412) -> ("error out"=w418:errorcluster, "State Send?"=w416:bool, "Modbus master out"=w417:refnum<class "Modbus Master.lvclass">)  [unwired: 5 in]
              }
            }
            n144 = Bundle By Name(cluster=w383, "Reference Hardware(s).TCP master instance"=w377, "Reference Hardware(s).VISA reference Port"=w376) -> (w382:T2)
            n145 = Bundle By Name(cluster=T12 {"Digital Output 1_I"=FALSE, "error"={"status"=FALSE, "code"=0, "source"=""}} ("Digital Output 1 (Reply Payload)"), "Digital Output 1_I"=w375, "error"=w374) -> (w385:T12)
            n146 = case shown="True" w386 {
              tunnel: w387 -> [_ w421]
              tunnel: w385 -> [_ w420]
              frame False {
              }
              frame True {
                n147 = Send Notification(notification=w420, notifier=w421) -> ()  [unwired: 1 in, 2 out]
              }
            }
          }
          frame "Digital Output 2" {
            # "Digital Output 2 to Hardware"
            n148 = Variant To Data(error in=w440, type=T7 {"Digital Output 2"=FALSE, "Wait Notifier"=refnum, "wait for reply"=FALSE} ("Digital Output 2 Argument"), Variant=w439) -> (data=w437:T7, error out=w428:errorcluster)
            n149 = Unbundle By Name(w432) -> ("Reference Hardware(s).TCP master instance"=w424:refnum<class "Modbus Master.lvclass">, "Reference Hardware(s).VISA reference Port"=w425:refnum<visa-resource-name>, "Comunication Hardware DAQ.Hardware"=w427:T10)
            n150 = Unbundle By Name(w437) -> ("Digital Output 2"=w426:bool, "Wait Notifier"=w436:refnum<notifier>, "wait for reply"=w435:bool)
            n151 = case shown="\"PLC Logo\"" w427 {
              tunnel: [FALSE ("State Send?") w451 w459 w465] -> w423
              tunnel: [w442 w450 w458 w461] -> w430
              tunnel: [w444 w449 w457 w467] -> w422
              tunnel: [w441 w448 w453 w466] -> w429
              tunnel: w428 -> [w444 w447 w456 w464]
              tunnel: w426 -> [_ w445 w455 w463]
              tunnel: w425 -> [w442 w446 w454 w461]
              tunnel: w424 -> [w441 w448 w453 w462]
              frame "DAQ9219", Default {
                # "No hay nada"
              }
              frame "Arduino" {
                n152 = call "Write Digital Output.vi"("error in (no error)"=w447, "State"=w445, "#Pin Digital Out"=enum16{"DO-0", "DO-1", "DO-2", "DO-3"}."DO-2", "VISA reference in"=w446) -> ("error out"=w449:errorcluster, "State dispare?"=w451:bool, "VISA reference out"=w450:refnum<visa-resource-name>)  [unwired: 5 in]
              }
              frame "Xpress Board" {
                n153 = call "Write Digital Output.vi"("error in (no error)"=w456, "State"=w455, "#Pin Digital Out"=enum16{"DO-0", "DO-1", "DO-2", "DO-3"}."DO-2", "VISA reference in"=w454) -> ("error out"=w457:errorcluster, "State dispare?"=w459:bool, "VISA reference out"=w458:refnum<visa-resource-name>)  [unwired: 5 in]
              }
              frame "PLC Logo" {
                n154 = call "Digital Output 0-10V.vi"("error in (no error)"=w464, "State"=w463, "#Pin 0-10V"=enum16{"DO-0", "DO-1", "DO-2", "DO-3"}."DO-2", "Modbus Master in"=w462) -> ("error out"=w467:errorcluster, "State Send?"=w465:bool, "Modbus master out"=w466:refnum<class "Modbus Master.lvclass">)  [unwired: 5 in]
              }
            }
            n155 = Bundle By Name(cluster=T13 {"Digital Output 2_I"=FALSE, "error"={"status"=FALSE, "code"=0, "source"=""}} ("Digital Output 2 (Reply Payload)"), "Digital Output 2_I"=w423, "error"=w422) -> (w434:T13)
            n156 = Bundle By Name(cluster=w432, "Reference Hardware(s).TCP master instance"=w429, "Reference Hardware(s).VISA reference Port"=w430) -> (w431:T2)
            n157 = case shown="True" w435 {
              tunnel: w436 -> [_ w470]
              tunnel: w434 -> [_ w469]
              frame False {
              }
              frame True {
                n158 = Send Notification(notification=w469, notifier=w470) -> ()  [unwired: 1 in, 2 out]
              }
            }
          }
          frame "Digital Output 3" {
            # "Digital Output 3 to Hardware"
            n159 = Variant To Data(error in=w489, type=T8 {"Digital Output 3"=FALSE, "Wait Notifier"=refnum, "wait for reply"=FALSE} ("Digital Output 3 Argument"), Variant=w488) -> (data=w486:T8, error out=w479:errorcluster)
            n160 = Unbundle By Name(w486) -> ("Digital Output 3"=w477:bool, "Wait Notifier"=w485:refnum<notifier>, "wait for reply"=w484:bool)
            n161 = Unbundle By Name(w481) -> ("Reference Hardware(s).TCP master instance"=w475:refnum<class "Modbus Master.lvclass">, "Reference Hardware(s).VISA reference Port"=w476:refnum<visa-resource-name>, "Comunication Hardware DAQ.Hardware"=w478:T10)
            n162 = case shown="\"DAQ9219\", Default" w478 {
              tunnel: [FALSE ("State Send?") w500 w508 w514] -> w472
              tunnel: [w493 w499 w507 w510] -> w473
              tunnel: [w490 w498 w506 w516] -> w471
              tunnel: [w492 w494 w502 w515] -> w474
              tunnel: w479 -> [w490 w497 w505 w513]
              tunnel: w477 -> [_ w495 w504 w512]
              tunnel: w476 -> [w493 w496 w503 w510]
              tunnel: w475 -> [w492 w494 w502 w511]
              frame "DAQ9219", Default {
                # "No hay nada"
              }
              frame "Arduino" {
                n163 = call "Write Digital Output.vi"("error in (no error)"=w497, "State"=w495, "#Pin Digital Out"=enum16{"DO-0", "DO-1", "DO-2", "DO-3"}."DO-0", "VISA reference in"=w496) -> ("error out"=w498:errorcluster, "State dispare?"=w500:bool, "VISA reference out"=w499:refnum<visa-resource-name>)  [unwired: 5 in]
              }
              frame "Xpress Board" {
                n164 = call "Write Digital Output.vi"("error in (no error)"=w505, "State"=w504, "#Pin Digital Out"=enum16{"DO-0", "DO-1", "DO-2", "DO-3"}."DO-0", "VISA reference in"=w503) -> ("error out"=w506:errorcluster, "State dispare?"=w508:bool, "VISA reference out"=w507:refnum<visa-resource-name>)  [unwired: 5 in]
              }
              frame "PLC Logo" {
                n165 = call "Digital Output 0-10V.vi"("error in (no error)"=w513, "State"=w512, "#Pin 0-10V"=enum16{"DO-0", "DO-1", "DO-2", "DO-3"}."DO-0", "Modbus Master in"=w511) -> ("error out"=w516:errorcluster, "State Send?"=w514:bool, "Modbus master out"=w515:refnum<class "Modbus Master.lvclass">)  [unwired: 5 in]
              }
            }
            n166 = Bundle By Name(cluster=T14 {"Digital Output 3_I"=FALSE, "error"={"status"=FALSE, "code"=0, "source"=""}} ("Digital Output 3 (Reply Payload)"), "Digital Output 3_I"=w472, "error"=w471) -> (w483:T14)
            n167 = Bundle By Name(cluster=w481, "Reference Hardware(s).TCP master instance"=w474, "Reference Hardware(s).VISA reference Port"=w473) -> (w480:T2)
            n168 = case shown="True" w484 {
              tunnel: w485 -> [_ w519]
              tunnel: w483 -> [_ w518]
              frame False {
              }
              frame True {
                n169 = Send Notification(notification=w518, notifier=w519) -> ()  [unwired: 1 in, 2 out]
              }
            }
          }
          frame "---Copy This Frame---" {
            # "Duplicate this frame when creating new messages.  Change this comment in the duplicated frame to describe this message."
            n170 = Merge Errors(w522) -> (w521:errorcluster)
          }
          frame "---Exit and Error Handling---" {
            # "Separator - The following cases handle errors and exit messages."
          }
          frame "Simulate MHL Error" {
            # "#DQMH_HowTo The 'Simulate MHL Error' button  illustrates how the MHL handles errors. This event is instructional in nature and can be removed."
            # "Simulate an error occurring at the MHL"
            n171 = call "Module Name--constant.vi"() -> ("Module Name"=w525:string)  [unwired: 11 in]
            n172 = xnode "Error Ring"("parameter 0"=w525) -> ("error out"=w527:errorcluster)
            n173 = Merge Errors(w529, w527) -> (w528:errorcluster)
          }
          frame "Error" {
            # "Error - Check the error message data and respond accordingly. This message is sent by the \"Error Handler\" VIs at the end of each loop in this application."
            n174 = property class="Module Admin"(reference=w539) -> ("Accessors:External Launch"=w538:bool)  [unwired: 1 in, 2 out]
            n175 = Variant To Data(error in=w546, type=errorcluster {"status"=FALSE, "code"=0, "source"=""} ("error constant"), Variant=w541) -> (data=w547:errorcluster, error out=w544:errorcluster)
            n176 = call "Error Reported.vi"("Error"=w547) -> ()  [unwired: 10 in, 1 out]
            n177 = case shown="False" w538 {
              tunnel: [w552 _] -> w543
              tunnel: w540 -> [w550 _]
              tunnel: w547 -> [w551 _]
              frame False {
                # "If the module is running standalone, then pop up an error dialog and call the \"Exit\" message."
                n178 = call <vilib>:"Simple Error Handler.vi"("error in (no error)"=w551) -> ()  [unwired: 4 in, 5 out]
                n179 = call-poly <vilib>:"Delacor_lib_QMH_Enqueue Message (poly).vi"("Priority Message? (F)"=TRUE, "Message"="Exit", "Message Queue in"=w550) -> ("error out"=w552:errorcluster)  [unwired: 7 in, 1 out]
              }
              frame True {
                # "If the module was launched externally, calling the Error Reported broadcast VI is the only action performed by the \"Error\" message. The module's caller can then process the error appropriately."
              }
            }
            n180 = Merge Errors(w544, w543) -> (w537:errorcluster)
            n181 = call <vilib>:"Simple Error Handler.vi"("error in (no error)"=w537) -> ()  [unwired: 4 in, 5 out]
          }
          frame "Exit" {
            w558 = FALSE ("PLC Logo")
            w563 = 91  # 91: not all Exit messages will have an argument
            w565 = TRUE  # Stop the VI
            # "Release the message queue reference"
            # "#CodeNeeded - Add any required cleanup code here"
            # "Exit - Exit the application."
            n182 = Variant To Data(error in=w571, type=T4 {"Origin"="", "Exit via Stop Module Req?"=FALSE, "Wait for Module to stop?"=FALSE} ("Stop Argument"), Variant=w564) -> (data=w561:T4, error out=w567:errorcluster)
            n183 = call <vilib>:"Clear Errors.vi"("error in (no error)"=w567, "specific error code to clear (0: all)"=w563) -> ("error out"=w570:errorcluster)  [unwired: 4 in, 1 out]
            n184 = control-ref of="This VI"() -> (w560:refnum<vi>)
            n185 = call-dynamic "Delacor_lib_QMH_Release Message Queue.vi"("error in"=w570, "Message Queue"=w566) -> ("error out"=w569:errorcluster)  [unwired: 9 in]
            n186 = call "Handle Exit.vi"("Stop Argument"=w561, "Admin in"=w559, "VI reference"=w560) -> ("error out"=w555:errorcluster)  [unwired: 7 in, 1 out]
            n187 = Unbundle By Name(w554) -> ("Reference Hardware(s).VISA reference Port"=w557:refnum<visa-resource-name>, "Reference Hardware(s).task out"=w556:refnum<k21>, "Reference Hardware(s).TCP master instance"=w553:refnum<class "Modbus Master.lvclass">)
            n188 = Merge Errors(w569, w555) -> (w568:errorcluster)
            n189 = local write "NI - 9219"(w558) -> ()
            n190 = local write "PLC Logo"(w558) -> ()
            n191 = local write "Xpress Board"(w558) -> ()
            n192 = local write "Arduino UNO"(w558) -> ()
            n193 = local write "Estado de conexión"(w558) -> ()
            n194 = call <vilib>:"DAQmx Clear Task.vi"("task in"=w556, "error in"=w555) -> ()  [unwired: 13 in, 1 out]
            n195 = call-dynamic "Close.vi"("error in (no error)"=w555, "Modbus master in"=w553) -> ()  [unwired: 9 in, 1 out]
            n196 = VISA Close(VISA resource name=w557, error in (no error)=w555) -> ()  [unwired: 1 out]
          }
          frame Default {
            # "'Default' case only runs if there is a message that isn't defined in any of the other cases.  Output a programming error."
            n197 = call "Module Name--constant.vi"() -> ("Module Name"=w572:string)  [unwired: 11 in]
            n198 = xnode "Error Ring"("parameter 0"=w573, "parameter 1"=w572) -> ("error out"=w577:errorcluster)
            n199 = Merge Errors(w575, w577) -> (w576:errorcluster)
          }
        }
        n200 = call-dynamic "Delacor_lib_QMH_Error Handler - Message Handling Loop.vi"("error in"=w122, "Message Queue in"=w112) -> ("dup error in"=w119:errorcluster)  [unwired: 8 in, 1 out]
      }
    }
    frame Error {
      # "Synchronize Caller Events.vi will inform Start Module.vi that the module has launched and will let the code calling Start Module.vi register for broadcasts and would permit the caller receive the broadcast that an error occurred at launch time."
      n201 = call-dynamic "Delacor_lib_QMH_Release Message Queue.vi"("error in"=w588, "Message Queue"=w586) -> ("error out"=w587:errorcluster)  [unwired: 9 in]
      n202 = call "Synchronize Caller Events.vi"("Singleton Module Admin in"=w589) -> ("error out"=w594:errorcluster)  [unwired: 9 in, 1 out]
      n203 = call "Module Name--constant.vi"() -> ("Module Name"=w592:string)  [unwired: 11 in]
      n204 = Format Into String(format string="An error occurred during initialization. %s is no longer running.", w592) -> (resulting string=w590:string)  [unwired: 2 in, 1 out]
      n205 = Merge Errors(w587, w594) -> (w595:errorcluster)
      n206 = call "Error Reported.vi"("Additional Information"=w590, "Error"=w595) -> ()  [unwired: 9 in, 1 out]
    }
  }
  n207 = Merge Errors(w14, w17) -> (w13:errorcluster)
  n208 = call "Close Module.vi"("error in (no error)"=w13, "Module Admin in"=w9) -> ("error out"=w15:errorcluster, "External Launch"=w2:bool, "Module Admin out"=w3:refnum<class "Delacor_lib_QMH_Module Admin.lvclass">)  [unwired: 7 in]
  n209 = Unregister For Events(event registration refnum=w8, error in=w15) -> (error out=w1:errorcluster)
  n210 = case "External Launch?" shown="True" w2 {
    tunnel: w1 -> [_ w596]
    frame False {
    }
    frame True {
      n211 = case shown="No Error" w596 {
        frame No Error {
          n212 = invoke class="VI" method="FP.Close"() -> ()  [unwired: 3 in, 3 out]
        }
        frame Error {
          n213 = invoke class="VI" method="FP.Open"("Activate"=TRUE ("Activate?")) -> ()  [unwired: 4 in, 5 out]
        }
      }
    }
  }
  n214 = call <vilib>:"Simple Error Handler.vi"("error in (no error)"=w1) -> ()  [unwired: 4 in, 5 out]
  n215 = local write "Module Admin"(w3) -> ()
